vi "Destroy.vi"(8 "Error In":errorcluster, 11 "Known Host":refnum<class "KnownHost.lvclass">) -> (0 "Error Out":errorcluster, 3 "SSH":refnum<class "SSH.lvclass">)   [LabVIEW 2018, in "Toolkit.lvlib" / "KnownHost.lvclass"]
uses:
  KnownHost.lvclass
  SSH/SSH.lvclass
  KnownHost.lvclass/KnownHost.ctl
  SSH/SSH.lvclass/SSH.ctl
  Toolkit.lvlib
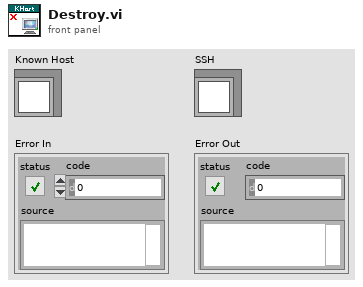
[diagram p1: front panel]
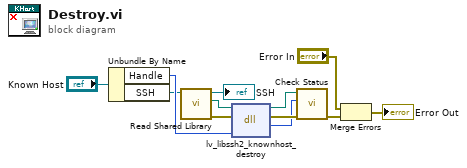
[diagram p0: block diagram]
diagram:
  n1 = Unbundle By Name("Known Host") -> ("Handle"=w10:u64, "SSH"=w4:refnum<class "SSH.lvclass">)
  n2 = call "Read Shared Library.vi"("SSH In"=w4) -> ("Error Out"=w2:errorcluster, "lv-libssh2 Shared Library"=w3:path, "SSH Out"=→"SSH":refnum<class "SSH.lvclass">)  [unwired: 8 in]
  n3 = dll-call lib="D:/Users/cfield/Code/Field R&D Services/SSH/LV-LIBSSH2/LabVIEW/trunk/src/Toolkit/Support/lv-libssh2.*" fn="lv_libssh2_knownhost_destroy"(path in=w3, error in=w2, "handle"=w10) -> (path out=w8:path, error out=w9:errorcluster, "status"=w7:i32)  [unwired: 2 in]
  n4 = call "Check Status.vi"("Error In"=w9, "Status"=w7, "lv-libssh2 Shared Library In"=w8) -> ("Error Out"=w6:errorcluster)  [unwired: 7 in, 1 out]
  n5 = Merge Errors("Error In", w6) -> (→"Error Out":errorcluster)
